vi "Release.vi"(8 "Error In":errorcluster, 11 "Listeners In":refnum<queue>[](array[refnum])) -> (0 "Error Out":errorcluster, 3 "Listeners Out":refnum<queue>[](array[refnum]))   [LabVIEW 2017, in "Toolkit.lvlib"]
uses:
  Toolkit.lvlib
  Controls/Statement.ctl
  Controls/Tag.ctl
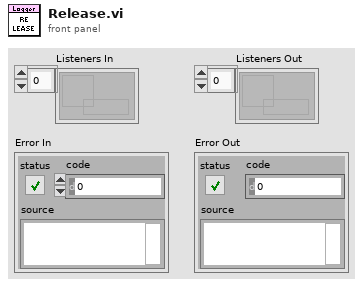
[diagram p1: front panel]
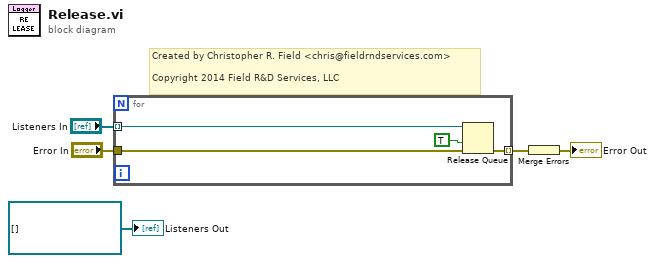
[diagram p0: block diagram]
diagram:
  # "Created by Christopher R. Field <chris@fieldrndservices.com>\n\nCopyright 2014 Field R&D Services, LLC"
  n1 = for {
    tunnel: "Listeners In" -> [w9] mode=indexing
    tunnel: "Error In" -> [w8]
    tunnel: [w7] -> w1 mode=indexing
    n2 = Release Queue(queue=w9, force destroy? (F)=TRUE, error in (no error)=w8) -> (error out=w7:errorcluster)  [unwired: 2 out]
  }
  n3 = Merge Errors(w1) -> (→"Error Out":errorcluster)
  "Listeners Out" <- refnum<queue>[] [] ("Listeners Out")
